vi "Read FPGA_Ctl.vi"(8 "error in":errorcluster, 11 "PAS Cell in":refnum<class "PAS Cell.lvclass">) -> (0 "error out":errorcluster, 2 "FPGA_Ctl":cluster{"Mod":T1, "Span":sgl, "f0":sgl} {"f0" format="%#_2g"}, 3 "PAS Cell out":refnum<class "PAS Cell.lvclass">)   [LabVIEW 2015, in "PAS Cell.lvclass"]
uses:
  PAS Cell.lvclass
  Main/Controls/Laser Modulation.ctl
  PAS Cell.lvclass/PAS Cell.ctl
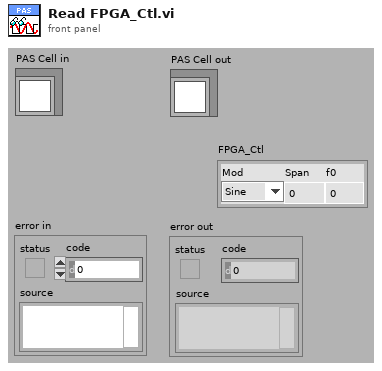
[diagram p1: front panel]
types:
  T1 = typedef "Laser Modulation.ctl" = enum8{"Sine", "Square"}
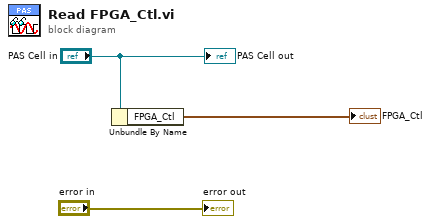
[diagram p0: block diagram]
diagram:
  n1 = Unbundle By Name("PAS Cell in") -> ("FPGA_Ctl"=→"FPGA_Ctl":cluster{"Mod":T1, "Span":sgl, "f0":sgl})
  "error out" <- "error in"
  "PAS Cell out" <- "PAS Cell in"
